vi "更新报表.vi"(3 "油动机名称":string, 4 "油动机试验路径":path, 5 "项目名称":string) -> ()   [LabVIEW 2013]
uses:
  <vilib>/Utility/config.llb/Read Key (String).vi
  <vilib>/Utility/config.llb/Write Key (String).vi
  <vilib>/Utility/config.llb/NI_LVConfig.lvlib
panel:
  in  "试验表格项":string[](array[string])=["活塞直径D", "活塞杆直径d", "工作行程Vh2.3", "超行程Oh1", "超行程Oh2", "位移传感器量程TS", "要求起始位2.4.2", "要求灵敏度2.4.2", "要求总行程Gh2.4.2", "理论F12.4.3", "理论F22.4.3", "理论摩擦力F2.4.3", "要求开关延时_开启2.4.5", "要求开关延时_关闭2.4.5", "要求开关延时_归零2.4.5", "要求延迟时间tv_2.4.5", "要求总关闭时间ts_2.4.5", "要求_终端速度_2.4.6", "阀门行程Vh"]
  in  "要求值表格项":string[](array[string])=["2.1_D_", "2.1_d0_", "2.1_vh_", "2.1_oh1_", "2.1_oh2_", "2.1_TS_", "2.4.2_起始位_", "2.4.2_灵敏度_", "2.4.2_总行程_", "2.4.3_F1_", "2.4.3_F2_", "2.4.3_F_", "2.4.5_OP_", "2.4.5_CL_", "2.4.5_DFT_", "2.4.5_tv_", "2.4.5_ts_", "2.4.6_EV_", "2.1_vh_"]
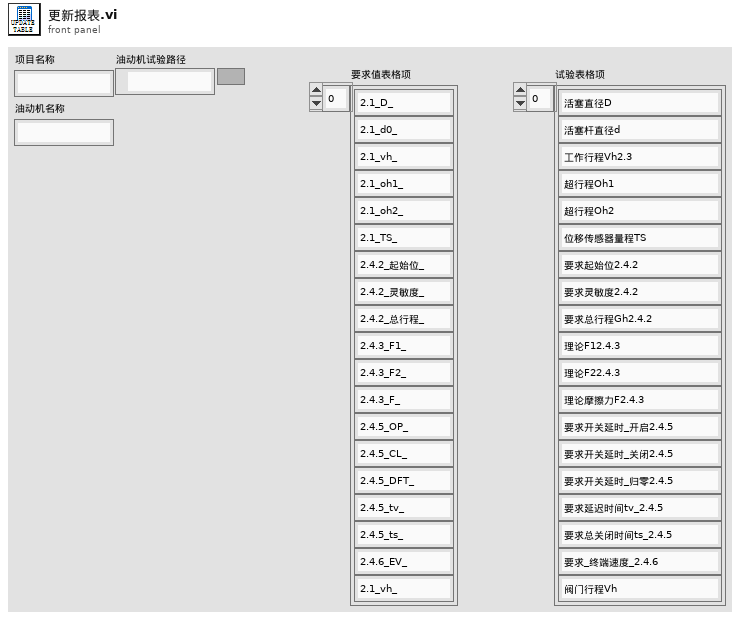
[diagram p1: front panel]
types:
  T1 = typedef "NI_LVConfig.lvlib/Config Data RefNum.ctl" = refnum<k1>
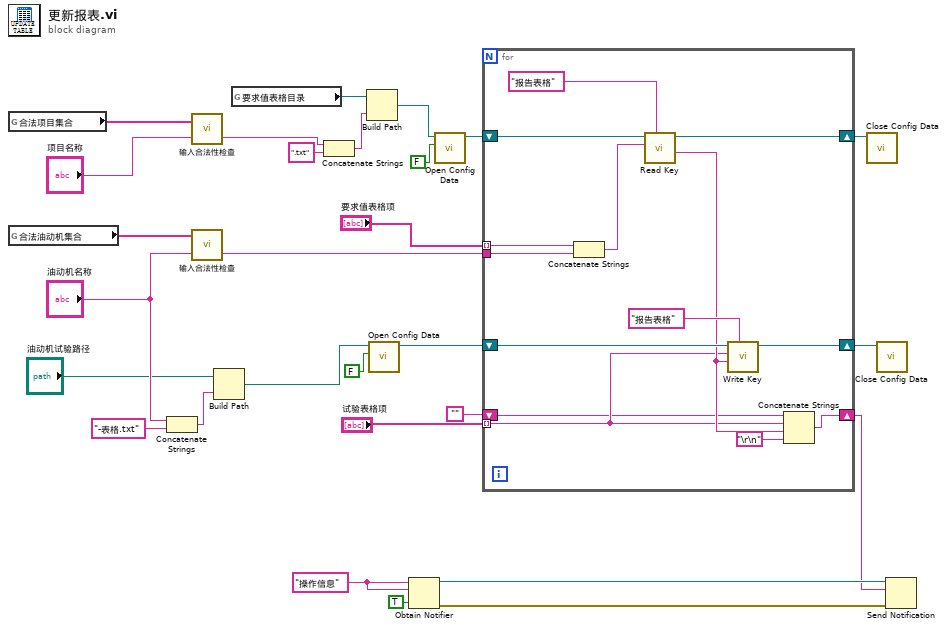
[diagram p0: block diagram]
diagram:
  w13 = "操作信息"
  n1 = global read "合法项目集合.vi" "合法项目集合"() -> (w23:string[])
  n2 = global read "合法油动机集合.vi" "合法油动机集合"() -> (w22:string[])
  n3 = Concatenate Strings("油动机名称", "-表格.txt" ("字符串")) -> (w8:string)
  n4 = call "输入合法性检查.vi"("被检查名称"="项目名称", "合法名称集合"=w23) -> ("合法名称"=w21:string)  [unwired: 1 out]
  n5 = call "输入合法性检查.vi"("被检查名称"="油动机名称", "合法名称集合"=w22) -> ("合法名称"=w20:string)  [unwired: 1 out]
  n6 = Build Path(base path="油动机试验路径", name or relative path=w8) -> (appended path=w7:path)
  n7 = global read "要求值表格目录.vi" "要求值表格目录"() -> (w24:path)
  n8 = Concatenate Strings(w21, ".txt" ("string")) -> (w25:string)
  n9 = Build Path(base path=w24, name or relative path=w25) -> (appended path=w28:path)
  n10 = call <vilib>:"Open Config Data.vi"("create file if necessary (T)"=FALSE, "configuration file path"=w7) -> ("refnum"=w17:T1)  [unwired: 7 in, 2 out]
  n11 = Obtain Notifier(name (unnamed)=w13, notification data type=w13, create if not found? (T)=TRUE) -> (notifier out=w12:refnum<notifier>, error out=w11:errorcluster)  [unwired: 1 in, 1 out]
  n12 = call <vilib>:"Open Config Data.vi"("create file if necessary (T)"=FALSE, "configuration file path"=w28) -> ("refnum"=w19:T1)  [unwired: 7 in, 2 out]
  n13 = for {
    tunnel: w20 -> [w42]
    shift-right: [w37] -> w15
    shift-left: w17 -> [w39]
    shift-right: [w38] -> w16
    shift-left: w19 -> [w41]
    tunnel: "试验表格项" -> [w34] mode=indexing
    tunnel: "要求值表格项" -> [w33] mode=indexing
    shift-right: [w30] -> w1
    shift-left: "" -> [w31]
    n14 = Concatenate Strings(w33, w42) -> (w40:string)
    n15 = call-poly <vilib>:"Read Key.vi"("section"="报告表格", "key"=w40, "refnum"=w41) -> ("value"=w35:string, "refnum out"=w38:T1)  [unwired: 5 in, 2 out]
    n16 = call-poly <vilib>:"Write Key.vi"("section"="报告表格", "value"=w35, "key"=w34, "refnum"=w39) -> ("refnum out"=w37:T1)  [unwired: 5 in, 2 out]
    n17 = Concatenate Strings(w31, w34, w35, "\r\n") -> (w30:string)
  }
  n18 = call <vilib>:"Close Config Data.vi"("refnum"=w16) -> ()  [unwired: 9 in, 2 out]
  n19 = call <vilib>:"Close Config Data.vi"("refnum"=w15) -> ()  [unwired: 9 in, 2 out]
  n20 = Send Notification(notification=w1, notifier=w12, error in (no error)=w11) -> ()  [unwired: 2 out]
